vi "get duplicate file name.vi"(11 "path list":string[](array[string])) -> (3 "Array":path[](array[path]))   [LabVIEW 2023]
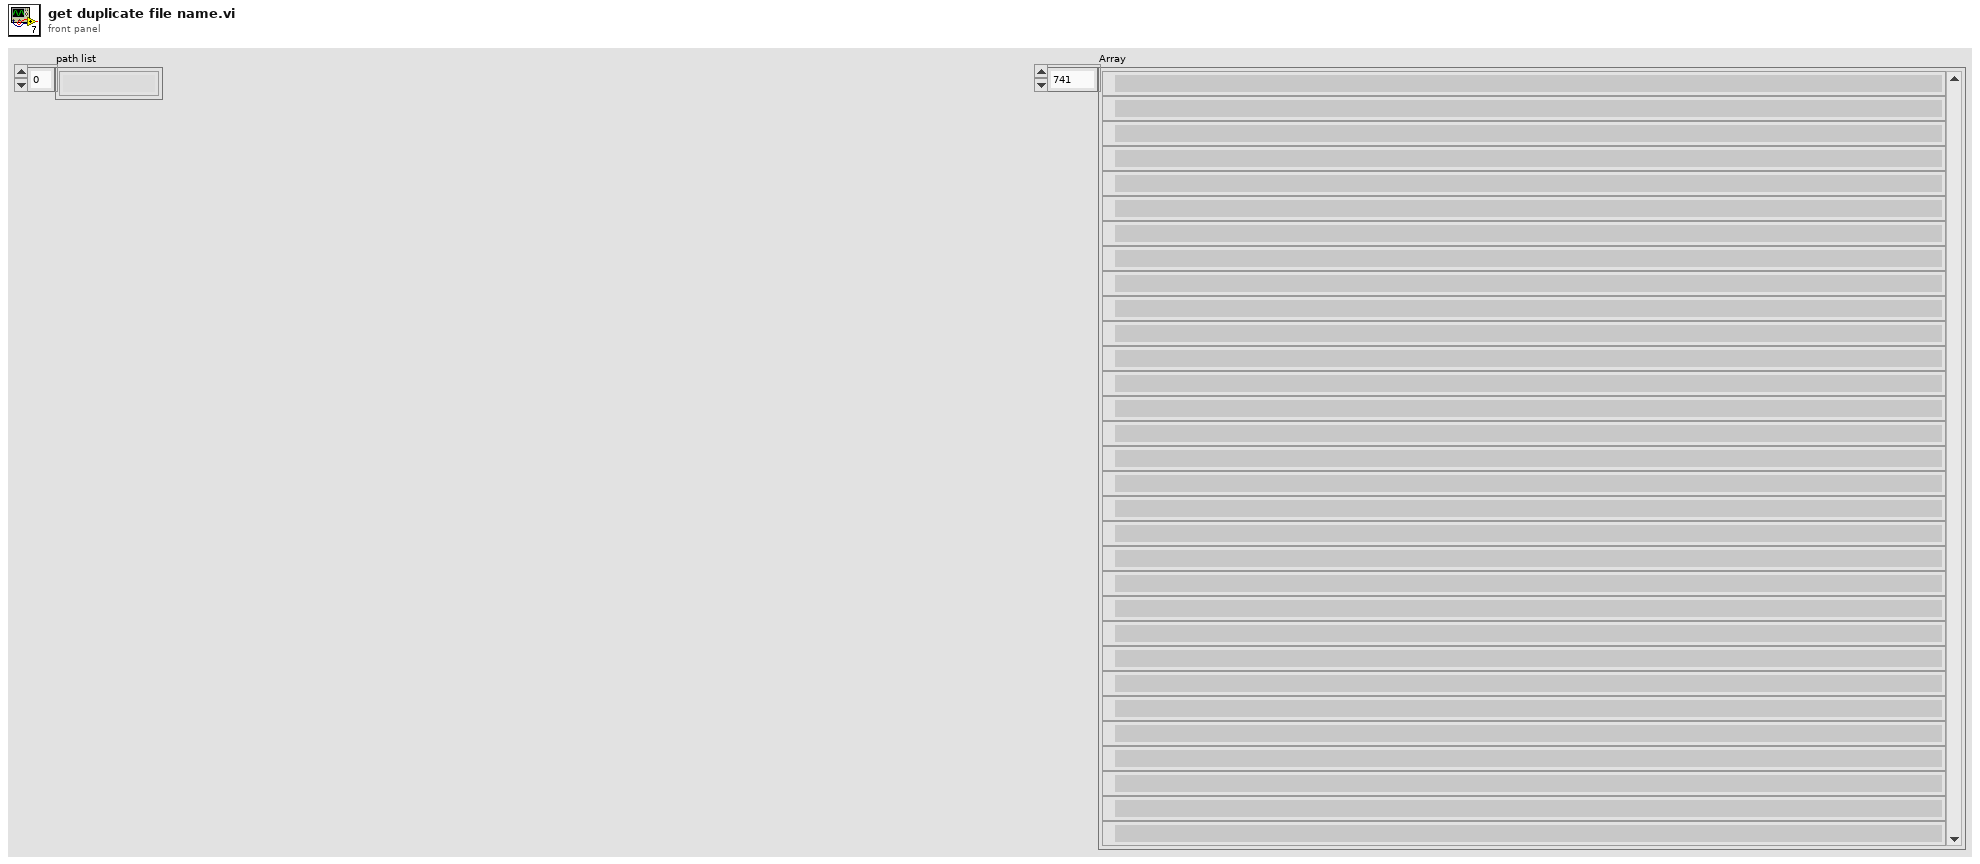
[diagram p1: front panel]
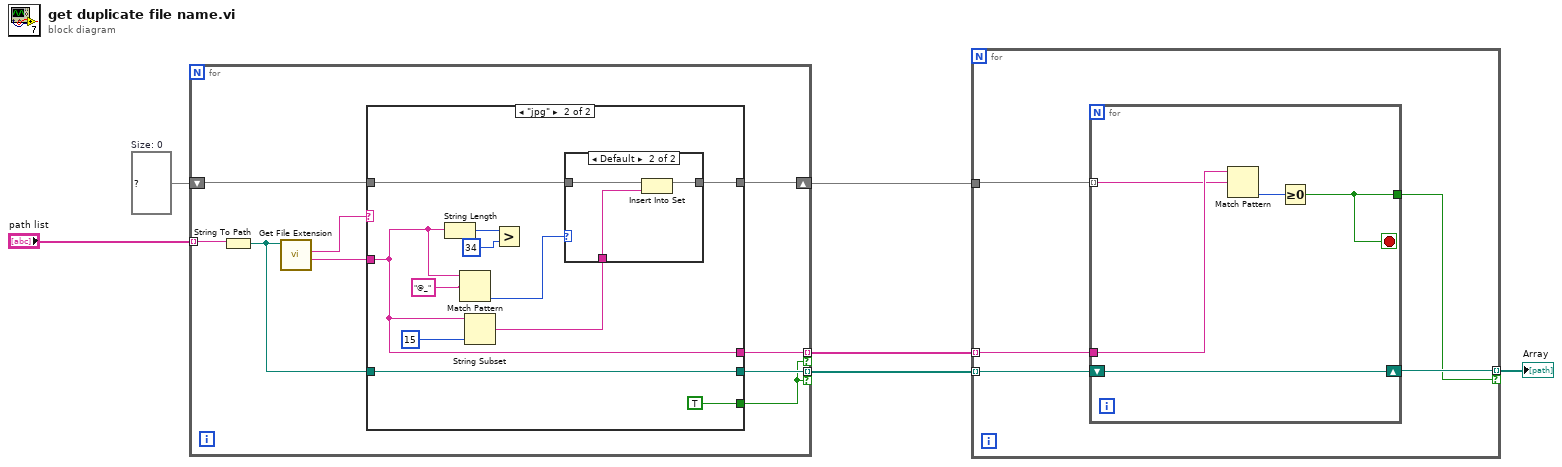
[diagram p0: block diagram]
diagram:
  w6 = set{string} {}  # Size: 0
  n1 = for {
    tunnel: "path list" -> [w15] mode=indexing
    shift-right: [w12] -> w2
    shift-left: w6 -> [w11]
    tunnel: [w10] -> w4 mode=indexing if=w7
    tunnel: [w8] -> w3 mode=indexing if=w7
    n2 = String To Path(string=w15) -> (path=w9:path)
    n3 = call <vilib>:"Get File Extension.vi"("file"=w9) -> ("filename without extension"=w13:string, "lowercase file extension"=w14:string)  [unwired: 6 in, 3 out]
    n4 = case shown="\"jpg\"" w14 {
      tunnel: w13 -> [_ w19]
      tunnel: [w16 w23] -> w12
      tunnel: w11 -> [w16 w22]
      tunnel: [_ w21] -> w10
      tunnel: w9 -> [_ w21]
      tunnel: [_ TRUE] -> w7
      tunnel: [_ w19] -> w8
      frame Default {
      }
      frame "jpg" {
        n5 = String Length(string=w19) -> (length=w26:i32)
        n6 = Match Pattern(string=w19, regular expression="@_") -> (offset past match=w17:i32)  [unwired: 1 in, 3 out]
        n7 = String Subset(string=w19, length (rest)=15 ("length (rest)")) -> (substring=w24:string)  [unwired: 1 in]
        n8 = Greater?(x=w26, y=34) -> ()  [unwired: 1 out]
        n9 = case shown="Default" w17 {
          tunnel: w24 -> [_ w31]
          tunnel: [w28 w30] -> w23
          tunnel: w22 -> [w28 w29]
          frame -1 {
          }
          frame Default {
            n10 = Insert Into Set(10:w31, 11:w29) -> (3:w30:set{string})  [unwired: 1 out]
          }
        }
      }
    }
  }
  n11 = for {
    tunnel: w4 -> [w33] mode=indexing
    tunnel: w3 -> [w35] mode=indexing
    tunnel: w2 -> [w36]
    tunnel: [w34] -> w1 mode=indexing if=w32
    n12 = for {
      tunnel: w36 -> [w40] mode=indexing
      tunnel: w35 -> [w41]
      shift-right: [w38] -> w34
      shift-left: w33 -> [w38]
      tunnel: [w37] -> w32
      stop <- w37 stop-if-true
      n13 = Match Pattern(string=w41, regular expression=w40) -> (offset past match=w39:i32)  [unwired: 1 in, 3 out]
      n14 = Greater Or Equal To 0?(x=w39) -> (x >= 0?=w37:bool)
    }
  }
  "Array" <- w1
